vi "Extract Routes.vi"(0 "Routes in":T1[](array[typedef]), 1 "From Location":cdb, 2 "Paths in":T4) -> (3 "Routes out":T1[](array[typedef]))   [LabVIEW 2020, in "AoC 2022.lvlib"]
uses:
  AoC 2022.lvlib
  Route.ctl
  Path.ctl
  Direction.ctl
  Paths.ctl
  702898fd-07ac-402b-8061-a8e75358be3e.vi
  0921e672-783f-4ae6-963c-78e0d4b74a45.vi
  702898fd-07ac-402b-8061-a8e75358be3e.vi/ff40df25-0e41-4205-825d-56c19dc320b6.vi
  0921e672-783f-4ae6-963c-78e0d4b74a45.vi/ff40df25-0e41-4205-825d-56c19dc320b6.vi
  <vilib>/Utility/Debug Log/Display.vi
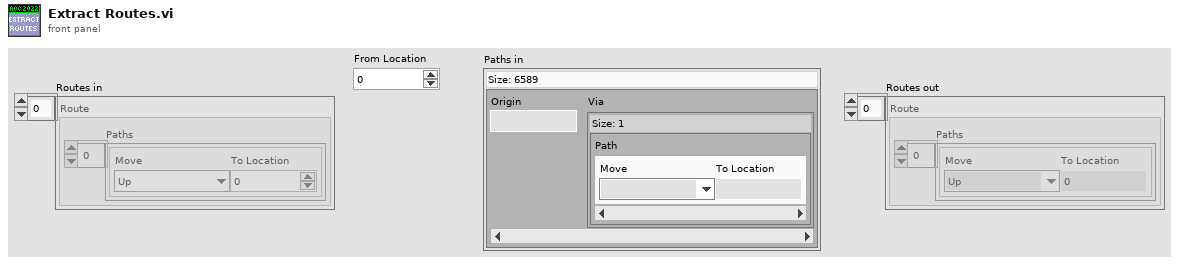
[diagram p1: front panel]
types:
  T1 = typedef "AoC 2022.lvlib/Route.ctl" = cluster{"Paths":T2[]}
  T2 = typedef "AoC 2022.lvlib/Path.ctl" = cluster{"Move":T3, "To Location":cdb}
  T3 = typedef "AoC 2022.lvlib/Direction.ctl" = enum16{"Up", "UpRight", "Right", "DownRight", "Down", "DownLeft", "Left", "UpLeft", "Stay"}
  T4 = typedef "AoC 2022.lvlib/Paths.ctl" = map{cdb, set{T2}}
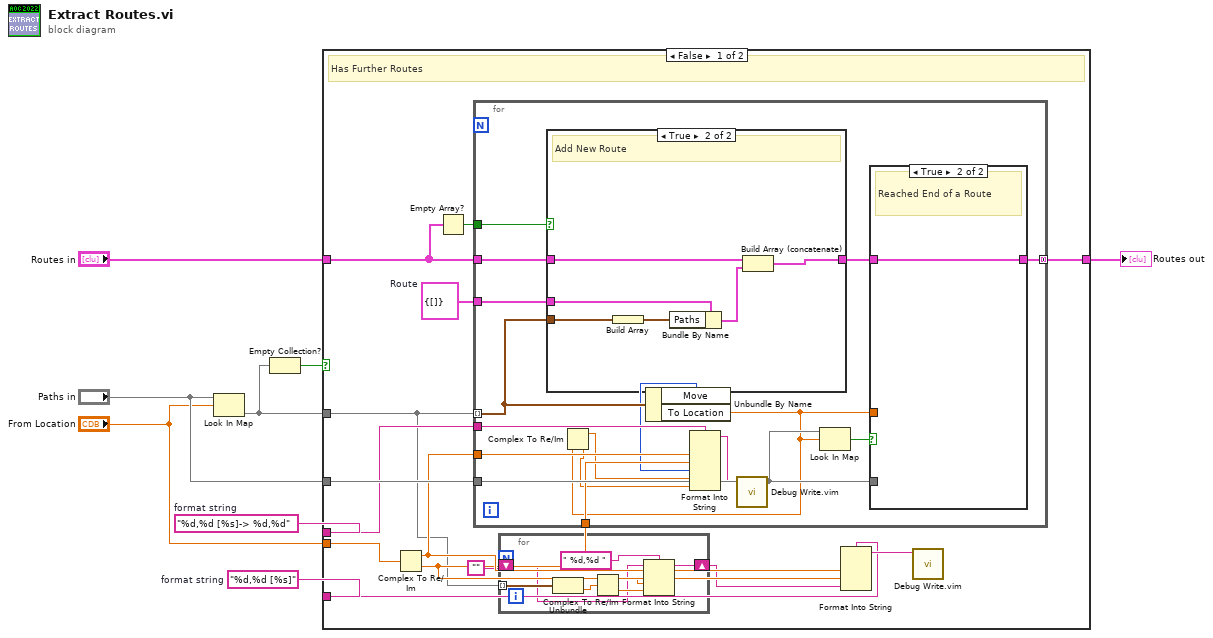
[diagram p0: block diagram]
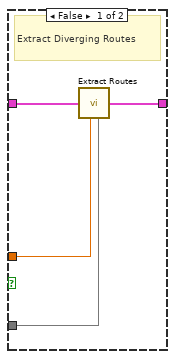
[diagram p2: hidden frame]
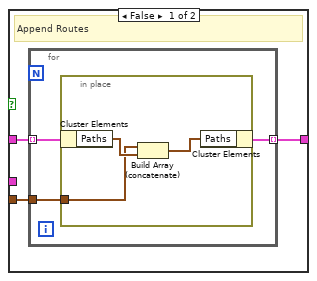
[diagram p3: hidden frame]
diagram:
  w1 = "%d,%d [%s]"  # format string
  w2 = "%d,%d [%s]-> %d,%d"  # format string
  n1 = Look In Map(map="Paths in", key="From Location") -> (value=w4:set{T2})  [unwired: 1 in, 1 out]
  n2 = Empty Collection?(1:w4) -> (0:w3:bool)
  n3 = case shown="False" w3 {
    tunnel: "Paths in" -> [w22 _]
    tunnel: "Routes in" -> [w20 w66]
    tunnel: [w19 w66] -> w6
    tunnel: w4 -> [w11 _]
    tunnel: "From Location" -> [w17 _]
    tunnel: w2 -> [w16 _]
    tunnel: w1 -> [w12 _]
    frame False {
      w18 = T1 {"Paths"=[]}  # Route
      # "Has Further Routes"
      n4 = Complex To Re/Im(x + iy=w17) -> (x=w14:dbl, y=w13:dbl)
      n5 = Empty Array?(array=w20) -> (empty?=w21:bool)
      n6 = for {
        tunnel: w11 -> [w38] mode=indexing
        tunnel: w22 -> [w41]
        tunnel: w20 -> [w45]
        tunnel: w21 -> [w44]
        tunnel: w18 -> [w43]
        tunnel: [w42] -> w19 mode=concatenating
        tunnel: w16 -> [w37]
        tunnel: w14 -> [w36]
        tunnel: w13 -> [w35]
        n7 = case shown="True" w44 {
          tunnel: w45 -> [w53 w63]
          tunnel: w38 -> [w52 w65]
          tunnel: w43 -> [_ w64]
          tunnel: [w51 w61] -> w39
          frame False {
            # "Append Routes"
            n8 = for {
              tunnel: w53 -> [w55] mode=indexing
              tunnel: w52 -> [w56]
              tunnel: [w54] -> w51 mode=indexing
              n9 = in-place {
                in-place-border: w56 -> [w57]
                n10 = in-place-cluster #1(w55) -> ("Paths"=w59:T2[])
                n11 = Build Array (concatenate)(w57, w59) -> (w58:T2[])
                n12 = in-place-cluster #1("Paths"=w58) -> (w54:T1)
              }
            }
          }
          frame True {
            # "Add New Route"
            n13 = Build Array(w65) -> (w60:T2[])
            n14 = Bundle By Name(cluster=w64, "Paths"=w60) -> (w62:T1)
            n15 = Build Array (concatenate)(w63, w62) -> (w61:T1[])
          }
        }
        n16 = Unbundle By Name(w38) -> ("Move"=w33:T3, "To Location"=w32:cdb)
        n17 = Complex To Re/Im(x + iy=w32) -> (x=w31:dbl, y=w30:dbl)
        n18 = Format Into String(format string=w37, w36, w35, w33, w31, w30) -> (resulting string=w34:string)  [unwired: 2 in, 1 out]
        n19 = call "Debug Write.vim"("value"=w34) -> ()  [unwired: 10 in, 1 out]
        n20 = Look In Map(map=w41, key=w32) -> (key not found?=w40:bool)  [unwired: 1 in, 1 out]
        n21 = case shown="True" w40 {
          tunnel: w32 -> [w49 _]
          tunnel: w39 -> [w48 w50]
          tunnel: [w47 w50] -> w42
          tunnel: w41 -> [w46 _]
          frame False {
            # "Extract Diverging Routes"
            n22 = call "Extract Routes.vi"("Routes in"=w48, "From Location"=w49, "Paths in"=w46) -> ("Routes out"=w47:T1[])
          }
          frame True {
            # "Reached End of a Route"
          }
        }
      }
      n23 = for {
        tunnel: w11 -> [w29] mode=indexing
        shift-right: [w24] -> w9
        shift-left: "" -> [w23]
        n24 = Unbundle(w29) -> ("To Location"=w28:cdb)  [unwired: 1 out]
        n25 = Complex To Re/Im(x + iy=w28) -> (x=w26:dbl, y=w27:dbl)
        n26 = Format Into String(format string=" %d,%d ", initial string=w23, w26, w27) -> (resulting string=w24:string)  [unwired: 1 in, 1 out]
      }
      n27 = Format Into String(format string=w12, w14, w13, w9) -> (resulting string=w15:string)  [unwired: 2 in, 1 out]
      n28 = call "Debug Write.vim"("value"=w15) -> ()  [unwired: 10 in, 1 out]
    }
    frame True {
      # "Has no Further Routes"
    }
  }
  "Routes out" <- w6
